vi "Queue References.vi"() -> ()   [LabVIEW 2015, in "myPAM.lvlib"]
uses:
  myPAM.lvlib
  Private TypeDefs/Message Queue Element.ctl
  Global TypeDefs/Registered Modules.ctl
  Private TypeDefs/Messages.ctl
panel:
  in  "Messaging Queue":refnum<queue>
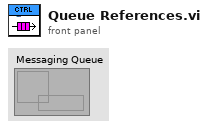
[diagram p1: front panel]
diagram:
